vi "test_MonoMoveToAndGetGratingPosition.vi"(0 "device selection":enum16{"monochromator", "CCD", "SCD"}(ring), 1 "Test should pass":bool=TRUE, 5 "set-up a connection":bool=TRUE, 9 "tear down connection":bool=TRUE, 11 "error in":errorcluster, 12 "Delay between send and receive [ms]":i32=100) -> (4 "first loop":i32, 6 "second loop":i32, 8 "third loop":i32, 10 "log-file path":path, 15 "error out":errorcluster)   [LabVIEW 2023]
uses:
  Classes/Mono/Monochromator.lvclass
  <vilib>/addons/_JKI Toolkits/Caraya/classes/Assert/Assert Equal Value and Type_Variant.vi
  <vilib>/addons/_JKI Toolkits/Caraya/classes/Assert/Assert Not Error.vi
  <vilib>/addons/_JKI Toolkits/Caraya/classes/Test/Test.lvclass
  <vilib>/addons/_JKI Toolkits/Caraya/classes/Assert/Assert.lvclass
  <vilib>/Hampel Software Engineering/HSE Logger/hse-logger.lvlib
panel:
  # "Connector Pane"
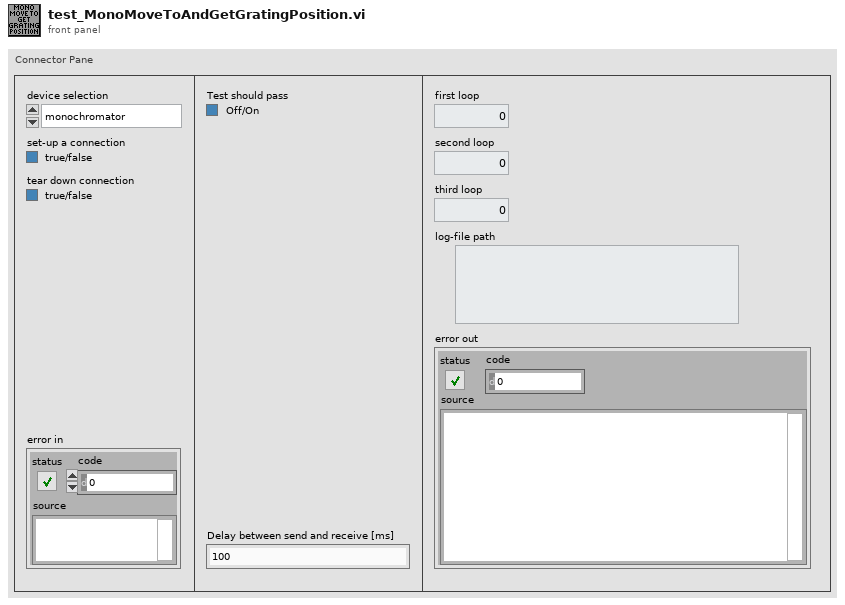
[diagram p1: front panel]
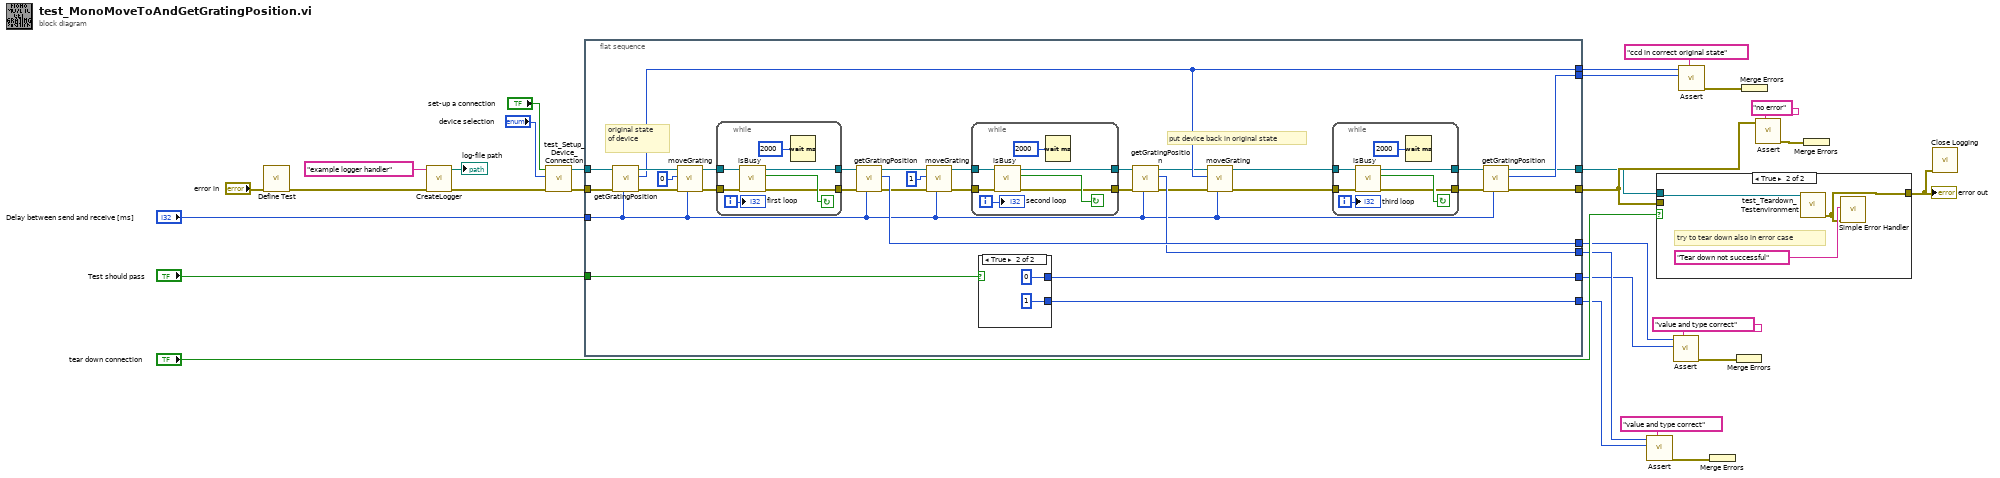
[diagram p0: block diagram]
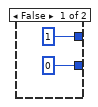
[diagram p2: hidden frame]
diagram:
  n1 = call <vilib>:"Define Test.vi"("error in (no error)"="error in") -> ("error out"=w3:errorcluster)  [unwired: 9 in, 1 out]
  n2 = call "CreateLogger.vi"("error in (no error)"=w3, "Handler Name"="example logger handler") -> ("error out"=w2:errorcluster, "log-file path"=→"log-file path":path)  [unwired: 8 in]
  n3 = call "test_Setup_Device_Connection.vi"("error in (no error)"=w2, "device selection"="device selection", "set-up a connection"="set-up a connection") -> ("error out"=w8:errorcluster, "Monochromator.lvclass"=w6:refnum<class "Monochromator.lvclass">)  [unwired: 5 in, 2 out]
  n4 = flat-sequence {
    tunnel: w8 -> [w57]
    tunnel: w6 -> [w58]
    tunnel: [w49] -> w20
    tunnel: "Test should pass" -> [w61]
    tunnel: [w50] -> w19
    tunnel: [w53] -> w18
    tunnel: [w60] -> w17
    tunnel: [w54] -> w16
    tunnel: [w59] -> w15
    tunnel: [w52] -> w12
    tunnel: [w51] -> w11
    tunnel: "Delay between send and receive [ms]" -> [w42]
    frame #0 {
      # "put device back in original state"
      # "original state of device"
      n5 = call "getGratingPosition.vi"("Delay between send and receive [ms]"=w42, "error in (no error)"=w57, "Monochromator in"=w58) -> ("error out"=w55:errorcluster, "position"=w52:i32, "Monochromator out"=w56:refnum<class "Monochromator.lvclass">)  [unwired: 6 in]
      n6 = call "moveGrating.vi"("Delay between send and receive [ms]"=w42, "error in (no error)"=w55, "position"=0, "Monochromator in"=w56) -> ("error out"=w44:errorcluster, "Monochromator out"=w46:refnum<class "Monochromator.lvclass">)  [unwired: 4 in, 2 out]
      n7 = while {
        tunnel: w46 -> [w73]
        tunnel: [w72] -> w45
        tunnel: w44 -> [w71]
        tunnel: [w70] -> w43
        i -> [w69]
        stop <- w75 continue-if-true
        n8 = call "isBusy.vi"("error in (no error)"=w71, "Monochromator in"=w73) -> ("error out"=w70:errorcluster, "Mono is busy?"=w75:bool, "Monochromator out"=w72:refnum<class "Monochromator.lvclass">)  [unwired: 7 in]
        n9 = Wait (ms)(milliseconds to wait=u32 2000) -> ()  [unwired: 1 out]
        "first loop" <- w69
      }
      n10 = call "getGratingPosition.vi"("Delay between send and receive [ms]"=w42, "error in (no error)"=w43, "Monochromator in"=w45) -> ("error out"=w34:errorcluster, "position"=w54:i32, "Monochromator out"=w35:refnum<class "Monochromator.lvclass">)  [unwired: 6 in]
      n11 = call "moveGrating.vi"("Delay between send and receive [ms]"=w42, "error in (no error)"=w34, "position"=1, "Monochromator in"=w35) -> ("error out"=w39:errorcluster, "Monochromator out"=w41:refnum<class "Monochromator.lvclass">)  [unwired: 4 in, 2 out]
      n12 = while {
        tunnel: w41 -> [w66]
        tunnel: [w65] -> w40
        tunnel: w39 -> [w64]
        tunnel: [w63] -> w38
        i -> [w62]
        stop <- w68 continue-if-true
        n13 = call "isBusy.vi"("error in (no error)"=w64, "Monochromator in"=w66) -> ("error out"=w63:errorcluster, "Mono is busy?"=w68:bool, "Monochromator out"=w65:refnum<class "Monochromator.lvclass">)  [unwired: 7 in]
        n14 = Wait (ms)(milliseconds to wait=u32 2000) -> ()  [unwired: 1 out]
        "second loop" <- w62
      }
      n15 = case shown="True" w61 {
        tunnel: [0 ("position") 1 ("position")] -> w60
        tunnel: [1 ("position") 0 ("position")] -> w59
        frame False {
        }
        frame True {
        }
      }
      n16 = call "getGratingPosition.vi"("Delay between send and receive [ms]"=w42, "error in (no error)"=w38, "Monochromator in"=w40) -> ("error out"=w36:errorcluster, "position"=w53:i32, "Monochromator out"=w37:refnum<class "Monochromator.lvclass">)  [unwired: 6 in]
      n17 = call "moveGrating.vi"("Delay between send and receive [ms]"=w42, "error in (no error)"=w36, "position"=w52, "Monochromator in"=w37) -> ("error out"=w31:errorcluster, "Monochromator out"=w33:refnum<class "Monochromator.lvclass">)  [unwired: 4 in, 2 out]
      n18 = while {
        tunnel: w33 -> [w84]
        tunnel: [w83] -> w32
        tunnel: w31 -> [w82]
        tunnel: [w81] -> w30
        i -> [w80]
        stop <- w86 continue-if-true
        n19 = call "isBusy.vi"("error in (no error)"=w82, "Monochromator in"=w84) -> ("error out"=w81:errorcluster, "Mono is busy?"=w86:bool, "Monochromator out"=w83:refnum<class "Monochromator.lvclass">)  [unwired: 7 in]
        n20 = Wait (ms)(milliseconds to wait=u32 2000) -> ()  [unwired: 1 out]
        "third loop" <- w80
      }
      n21 = call "getGratingPosition.vi"("Delay between send and receive [ms]"=w42, "error in (no error)"=w30, "Monochromator in"=w32) -> ("error out"=w49:errorcluster, "position"=w51:i32, "Monochromator out"=w50:refnum<class "Monochromator.lvclass">)  [unwired: 6 in]
    }
  }
  n22 = call-poly <vilib>:"Assert.vi"("Label"="value and type correct" ("Label (VI Title)"), "Y"=w17, "X"=w18) -> ("error out"=w28:errorcluster)  [unwired: 7 in, 1 out]
  n23 = case shown="True" "tear down connection" {
    tunnel: w19 -> [_ w89]
    tunnel: [w87 w88] -> w1
    tunnel: w20 -> [w87 _]
    frame False {
    }
    frame True {
      # "try to tear down also in error case"
      n24 = call "test_Teardown_Testenvironment.vi"("GenericDevice.lvclass"=w89) -> ("error out"=w88:errorcluster)  [unwired: 9 in, 1 out]
      n25 = call <vilib>:"Simple Error Handler.vi"("error source (\" \")"="Tear down not successful" ("error source (\" \")"), "error in (no error)"=w88) -> ()  [unwired: 3 in, 5 out]
    }
  }
  "error out" <- w1
  n26 = call-poly <vilib>:"Assert.vi"("Label"="value and type correct" ("Label (VI Title)"), "Y"=w15, "X"=w16) -> ("error out"=w27:errorcluster)  [unwired: 7 in, 1 out]
  n27 = call-poly <vilib>:"Assert.vi"("Label"="ccd in correct original state" ("Label (VI Title)"), "Y"=w11, "X"=w12) -> ("error out"=w14:errorcluster)  [unwired: 7 in, 1 out]
  n28 = Merge Errors(w28) -> ()  [unwired: 1 out]
  n29 = Merge Errors(w27) -> ()  [unwired: 1 out]
  n30 = Merge Errors(w14) -> ()  [unwired: 1 out]
  n31 = call-poly <vilib>:"Assert.vi"("Label"="no error" ("Label (VI Title)"), "Not Error?"=w20) -> ("error out"=w22:errorcluster)  [unwired: 8 in, 1 out]
  n32 = Merge Errors(w22) -> ()  [unwired: 1 out]
  n33 = call <vilib>:"Close Logging.vi"("error in"=w1) -> ()  [unwired: 10 in, 1 out]
